vi "Fetch Data.vi"(6 "wait for reply (T)":bool=TRUE, 7 "Data Results":refnum<vi>, 8 "error in":errorcluster, 9 "Start Time":timestamp, 10 "End Time":timestamp) -> (0 "error out":errorcluster, 1 "timed out?":bool, 3 "Reply Payload":T1)   [LabVIEW 2020, in "DataBase.lvlib"]
doc: "Update, save all to the SQlite DB\n_____\nCreated using Delacor QMH Event Scripter 6.0.0.121."
uses:
  DataBase.lvlib
  Fetch Data Argument--cluster.ctl
  Fetch Data (Reply Payload)--cluster.ctl
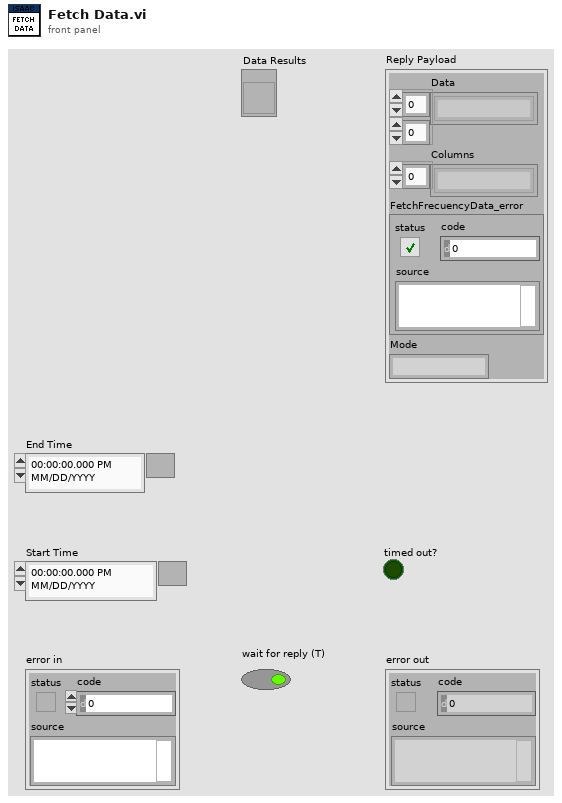
[diagram p1: front panel]
types:
  T1 = cluster{"Data":string[][], "Columns":string[], "FetchFrecuencyData_error":errorcluster, "Mode":string}
  T2 = typedef "DataBase.lvlib/Fetch Data Argument--cluster.ctl" = cluster{"End Time":timestamp, "Start Time":timestamp, "Data Results":refnum<vi>, "Wait Notifier":refnum<notifier>, "wait for reply":bool}
  T3 = typedef "DataBase.lvlib/Request Events--cluster.ctl" = cluster{"Stop Module":refnum<user-event>, "Show Panel":refnum<user-event>, "Hide Panel":refnum<user-event>, "Get Module Execution Status":refnum<user-event>, "Show Diagram":refnum<user-event>, "Fetch Data":refnum<user-event>}
  T4 = typedef "DataBase.lvlib/Fetch Data (Reply Payload)--cluster.ctl" = cluster{"Reply Payload":cluster{"Data":string[][], "Columns":string[], "FetchFrecuencyData_error":errorcluster}}
  T5 = cluster{"Data":string[][], "Columns":string[], "FetchFrecuencyData_error":errorcluster}
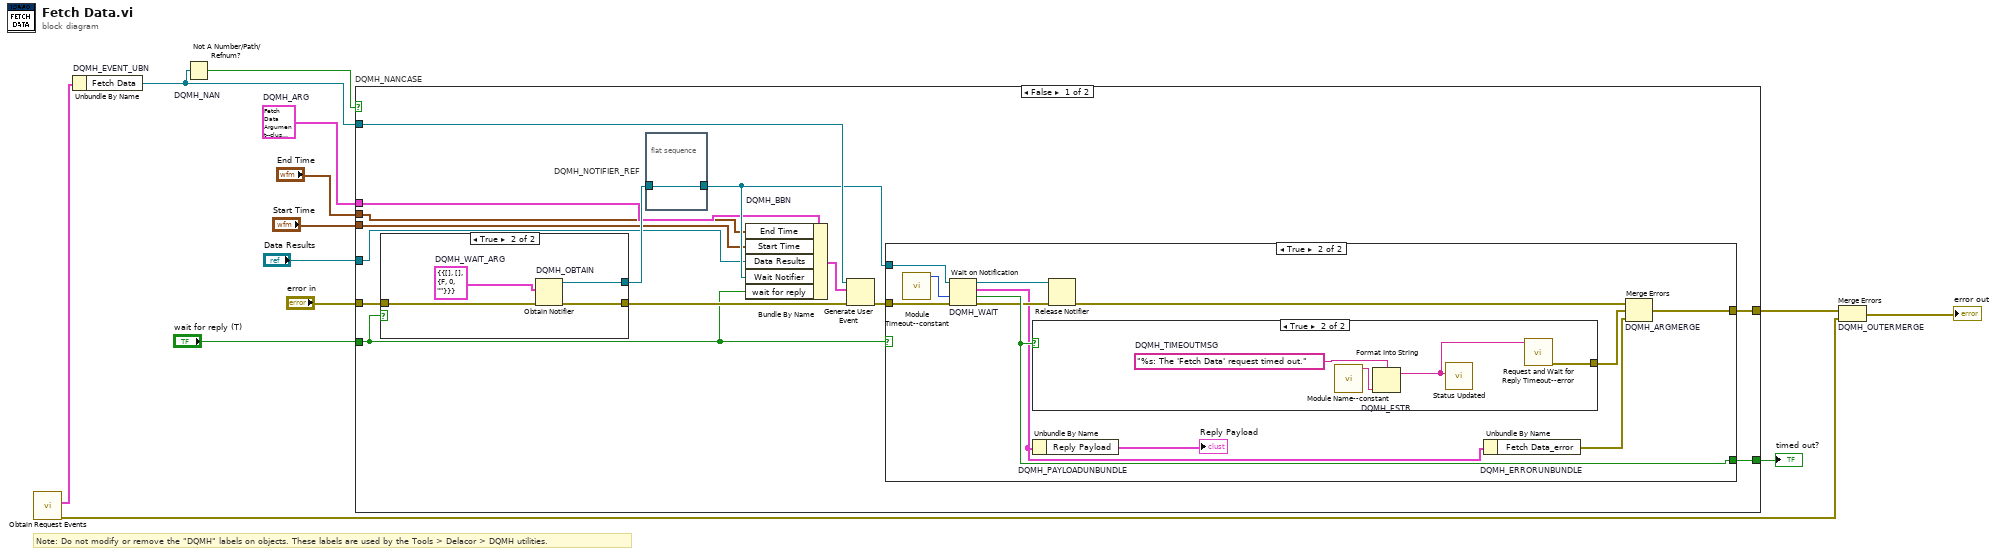
[diagram p0: block diagram]
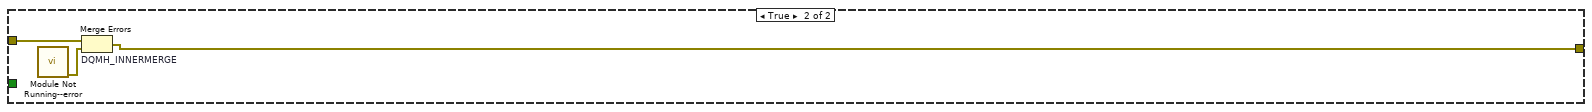
[diagram p5: hidden frame]
diagram:
  w7 = T2 {"End Time"=timestamp(0 s since 1904-01-01), "Start Time"=timestamp(0 s since 1904-01-01), "Data Results"=refnum, "Wait Notifier"=refnum, "wait for reply"=FALSE}  # DQMH_ARG
  # "Note: Do not modify or remove the \"DQMH\" labels on objects. These labels are used by the Tools > Delacor > DQMH utilities."
  n1 = call "Obtain Request Events.vi"() -> ("error out"=w2:errorcluster, "DataBase Request Events"=w1:T3)  [unwired: 10 in]
  n2 = Unbundle By Name "DQMH_EVENT_UBN"(w1) -> ("Fetch Data"=w11:refnum<user-event>)
  n3 = Not A Number/Path/Refnum? "DQMH_NAN"(number/path/refnum=w11) -> (NaN/Path/Refnum?=w10:bool)
  n4 = case "DQMH_NANCASE" shown="False" w10 {
    tunnel: "error in" -> [w27 w53]
    tunnel: w11 -> [w25 _]
    tunnel: [w22 w52] -> w8
    tunnel: [w23 _] -> w9
    tunnel: w7 -> [w18 _]
    tunnel: "End Time" -> [w17 _]
    tunnel: "Start Time" -> [w16 _]
    tunnel: "Data Results" -> [w15 _]
    tunnel: "wait for reply (T)" -> [w14 _]
    frame False {
      n5 = case shown="True" w14 {
        tunnel: w27 -> [w46 w50]
        tunnel: [w46 w49] -> w24
        tunnel: [_ w47] -> w20
        frame False {
        }
        frame True {
          w48 = T4 {"Reply Payload"={"Data"=[], "Columns"=[], "FetchFrecuencyData_error"={"status"=FALSE, "code"=0, "source"=""}}}  # DQMH_WAIT_ARG
          n6 = Obtain Notifier "DQMH_OBTAIN"(notification data type=w48, error in (no error)=w50) -> (notifier out=w47:refnum<notifier>, error out=w49:errorcluster)  [unwired: 2 in, 1 out]
        }
      }
      n7 = flat-sequence "DQMH_NOTIFIER_REF" {
        tunnel: w20 -> [w28]
        tunnel: [w28] -> w19
        frame #0 {
        }
      }
      n8 = Bundle By Name "DQMH_BBN"(cluster=w18, "End Time"=w17, "Start Time"=w16, "Data Results"=w15, "Wait Notifier"=w19, "wait for reply"=w14) -> (w21:T2)
      n9 = Generate User Event(user event=w25, event data cluster=w21, error in=w24) -> (error out=w26:errorcluster)  [unwired: 1 in, 1 out]
      n10 = case shown="True" w14 {
        tunnel: w26 -> [w29 w41]
        tunnel: w19 -> [_ w40]
        tunnel: [_ w38] -> w23
        tunnel: [w29 w37] -> w22
        frame False {
        }
        frame True {
          n11 = call "Module Timeout--constant.vi"() -> ("Module Timeout"=w31:i32)  [unwired: 11 in]
          n12 = Wait on Notification "DQMH_WAIT"(notifier=w40, timeout in ms (-1)=w31, error in (no error)=w41) -> (notifier out=w39:refnum<notifier>, notification=w32:T4, timed out?=w38:bool, error out=w36:errorcluster)  [unwired: 1 in]
          n13 = case shown="True" w38 {
            tunnel: [_ w43] -> w33
            frame False {
            }
            frame True {
              w45 = "%s: The 'Fetch Data' request timed out."  # DQMH_TIMEOUTMSG
              n14 = call "Module Name--constant.vi"() -> ("Module Name"=w42:string)  [unwired: 11 in]
              n15 = Format Into String "DQMH_FSTR"(format string=w45, w42) -> (resulting string=w44:string)  [unwired: 2 in, 1 out]
              n16 = call "Status Updated.vi"("Status"=w44) -> ()  [unwired: 10 in, 1 out]
              n17 = call "Request and Wait for Reply Timeout--error.vi"("Error Message"=w44) -> ("error out"=w43:errorcluster)  [unwired: 10 in]
            }
          }
          n18 = Unbundle By Name "DQMH_PAYLOADUNBUNDLE"(w32) -> ("Reply Payload"=→"Reply Payload":T5)
          n19 = Release Notifier(notifier=w39, error in (no error)=w36) -> (error out=w35:errorcluster)  [unwired: 1 in, 2 out]
          n20 = Unbundle By Name "DQMH_ERRORUNBUNDLE"(w32) -> ("Fetch Data_error"=w34:errorcluster)
          n21 = Merge Errors "DQMH_ARGMERGE"(w35, w33, w34) -> (w37:errorcluster)
        }
      }
    }
    frame True {
      n22 = call "Module Not Running--error.vi"() -> ("error out"=w51:errorcluster)  [unwired: 11 in]
      n23 = Merge Errors "DQMH_INNERMERGE"(w53, w51) -> (w52:errorcluster)
    }
  }
  "timed out?" <- w9
  n24 = Merge Errors "DQMH_OUTERMERGE"(w8, w2) -> (→"error out":errorcluster)
